vi "Lockstep Move at Velocity (Polymorphic).vi"   [LabVIEW 2013, in "Zaber A Series.lvlib"]
doc: "Moves a lockstep group at a specified velocity. Velocity is specified in native device speed units; check your device manual for the conversion factor or use the Conver Velocity Units to Device Units VI.\n\nConstant velocity movement stops when the stage reaches the end of its travel, a stop command is sent, or a new movement command is sent.\n\nThis VI requires that the Initialize VI has been called with the same serial port and that the lockstep group has already been enabled. \n\nNote: See the Device Lookup control for the microstep size of your model, or check on the product specifications page for the product on www.zaber.com."
uses:
  Zaber A Series.lvlib
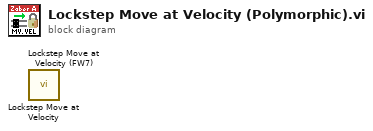
[diagram p0: block diagram]
diagram:
  n1 = call "Lockstep Move at Velocity.vi"() -> ()  [unwired: 10 in, 2 out]
  n2 = call "Lockstep Move at Velocity (FW7).vi"() -> ()  [unwired: 10 in, 2 out]
